vi "CreateDataTable.vi"(8 "error in (no error)":errorcluster, 9 "String Data":string[][](array[string]), 10 "Columns":refnum<class "GridColumn.lvclass">[](array[class]), 11 "DataTable in":refnum<class "DataTable.lvclass">) -> (0 "error out":errorcluster, 3 "DataTable out":refnum<class "DataTable.lvclass">)   [LabVIEW 2014, in "DataTable.lvclass"]
uses:
  DataTable.lvclass
  GridColumn/GridColumn.lvclass
  DataTable.lvclass/DataTable.ctl
  System.Data
  GridColumn/GridColumn.lvclass/GridColumn.ctl
  GridColumn/Read datatype.vi
  GridColumn/Read Params.vi
  GridColumn/Read Name.vi
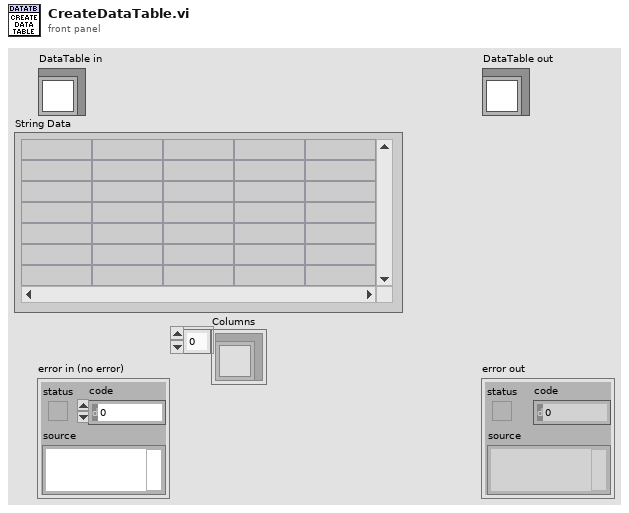
[diagram p1: front panel]
types:
  T1 = enum16{"string", "image", "check", "numeric", "timestamp", "button", "combo"}
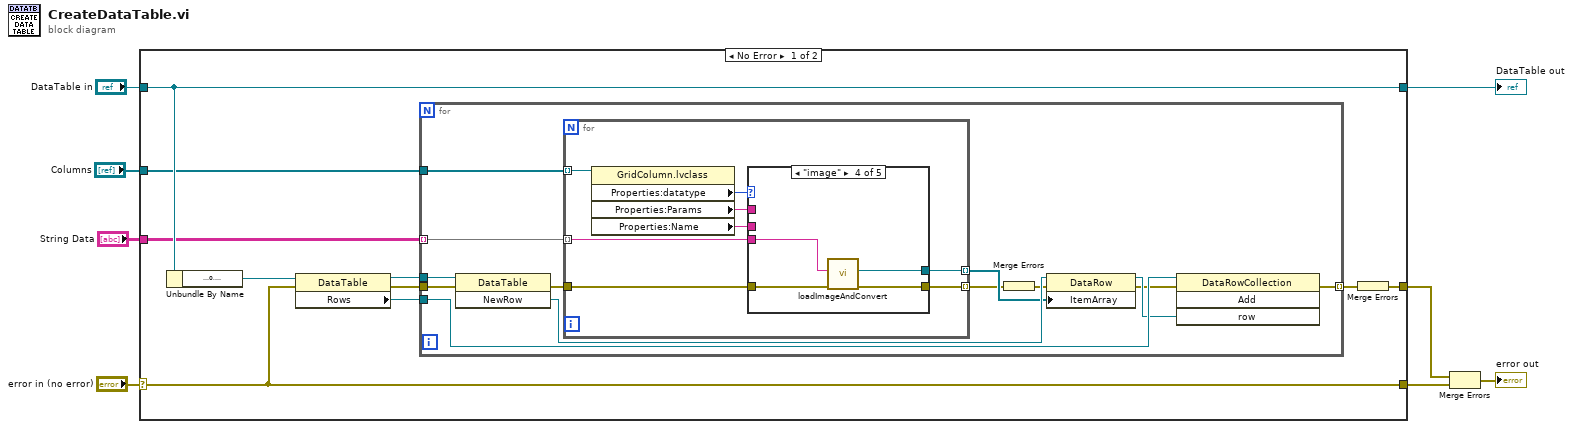
[diagram p0: block diagram]
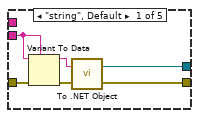
[diagram p2: hidden frame]
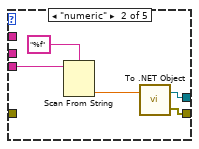
[diagram p3: hidden frame]
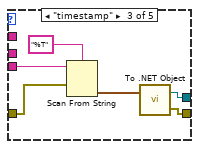
[diagram p4: hidden frame]
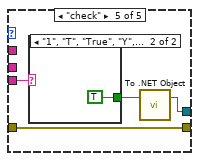
[diagram p5: hidden frame]
diagram:
  n1 = case shown="No Error" "error in (no error)" {
    selector: "error in (no error)" -> [w14 w67]
    tunnel: [w14 w67] -> w7
    tunnel: [w15 w66] -> w5
    tunnel: "DataTable in" -> [w15 w66]
    tunnel: "String Data" -> [w13 _]
    tunnel: "Columns" -> [w12 _]
    tunnel: [w9 _] -> w1
    frame No Error {
      n2 = Unbundle By Name(w15) -> ("DataTable"=w11:refnum<k24>)
      n3 = property class="DataTable"(reference=w11, error in=w14) -> (reference out=w10:refnum<k24>, error out=w18:errorcluster, "Rows"=w17:refnum<k24>)
      n4 = for {
        tunnel: w17 -> [w30]
        tunnel: w10 -> [w31]
        tunnel: [w29] -> w16 mode=indexing
        tunnel: w13 -> [w28] mode=indexing
        tunnel: w18 -> [w20]
        tunnel: w12 -> [w19]
        n5 = invoke class="DataTable" method="NewRow"(reference=w31, error in=w20) -> (error out=w27:errorcluster, "NewRow"=w26:refnum<k24>)  [unwired: 1 in, 1 out]
        n6 = for {
          tunnel: w28 -> [w39] mode=indexing
          tunnel: [w38] -> w24 mode=indexing
          tunnel: w27 -> [w37]
          tunnel: [w36] -> w23 mode=indexing
          tunnel: w19 -> [w35] mode=indexing
          n7 = property class="GridColumn.lvclass"(reference=w35) -> ("Properties:datatype"=w34:T1, "Properties:Params"=w33:string, "Properties:Name"=w32:string)  [unwired: 1 in, 2 out]
          n8 = case shown="\"image\"" w34 {
            tunnel: w39 -> [w41 w48 w54 w60 w62]
            tunnel: [w40 w49 w55 w59 w63] -> w38
            tunnel: w37 -> [w44 _ w52 w58 w64]
            tunnel: [w42 w50 w56 w57 w64] -> w36
            tunnel: w33 -> [_ _ _ _ _]
            tunnel: w32 -> [_ _ _ _ _]
            frame "string", Default {
              n9 = Variant To Data(error in=w44, type=w41, Variant=w41) -> (data=w45:string, error out=w43:errorcluster)
              n10 = call <vilib>:"To .NET Object.vi"("error in (no error)"=w43, "anything"=w45) -> ("error out"=w42:errorcluster, ".NET object"=w40:refnum<k24>)
            }
            frame "numeric" {
              n11 = Scan From String(format string="%f", input string=w48) -> (output 1=w46:dbl)  [unwired: 3 in, 3 out]
              n12 = call <vilib>:"To .NET Object.vi"("anything"=w46) -> ("error out"=w50:errorcluster, ".NET object"=w49:refnum<k24>)  [unwired: 1 in]
            }
            frame "timestamp" {
              n13 = Scan From String(format string="%T", input string=w54, error in=w52) -> (output 1=w51:timestamp)  [unwired: 2 in, 3 out]
              n14 = call <vilib>:"To .NET Object.vi"("anything"=w51) -> ("error out"=w56:errorcluster, ".NET object"=w55:refnum<k24>)  [unwired: 1 in]
            }
            frame "image" {
              n15 = call "loadImageAndConvert.vi"("error in (no error)"=w58, "name or relative path"=w60) -> ("error out"=w57:errorcluster, ".NET object"=w59:refnum<k24>)  [unwired: 8 in]
            }
            frame "check" {
              n16 = case shown="\"1\", \"T\", \"True\", \"Y\", \"Yes\"" w62 {
                tunnel: [_ TRUE] -> w61
                frame Default {
                }
                frame "1", "T", "True", "Y", "Yes" {
                }
              }
              n17 = call <vilib>:"To .NET Object.vi"("anything"=w61) -> (".NET object"=w63:refnum<k24>)  [unwired: 1 in, 1 out]
            }
          }
        }
        n18 = Merge Errors(w23) -> (w22:errorcluster)
        n19 = property class="DataRow"(reference=w26, error in=w22, "ItemArray"=w24) -> (reference out=w25:refnum<k24>, error out=w21:errorcluster)
        n20 = invoke class="DataRowCollection" method="Add"(reference=w30, error in=w21, "row"=w25) -> (error out=w29:errorcluster)  [unwired: 1 in, 3 out]
      }
      n21 = Merge Errors(w16) -> (w9:errorcluster)
    }
    frame Error {
    }
  }
  "DataTable out" <- w5
  n22 = Merge Errors(w1, w7) -> (→"error out":errorcluster)
